vi "Desktop Main.vi"() -> ()   [LabVIEW 2021]
doc: "Demonstrates how to use User Datagram Protocol (UDP) to send data to the myRIO target."
panel:
  in  "LED":bool[](array[boolean])=[FALSE, FALSE, FALSE, FALSE]
  out "error out":errorcluster
  in  "Stop":bool
  in  "Target IP Address":string="172.22.11.2"
  # "Overview: Demonstrates how to use User Datagram Protocol (UDP) to send data to the myRIO target.\nInstructions:\n1. Verify if the value of Target IP Address is correct. If not, specify the correct value.\n2. Run this VI.\n3. Open RT Main.vi and follow its front panel instructions.\n4. Change the value of LED on this VI and observe the value of LED Status on RT Main.vi.\n5. Click Stop to stop this VI."
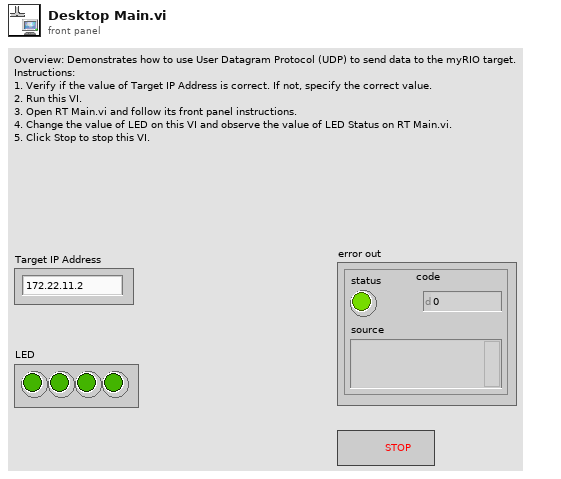
[diagram p1: front panel]
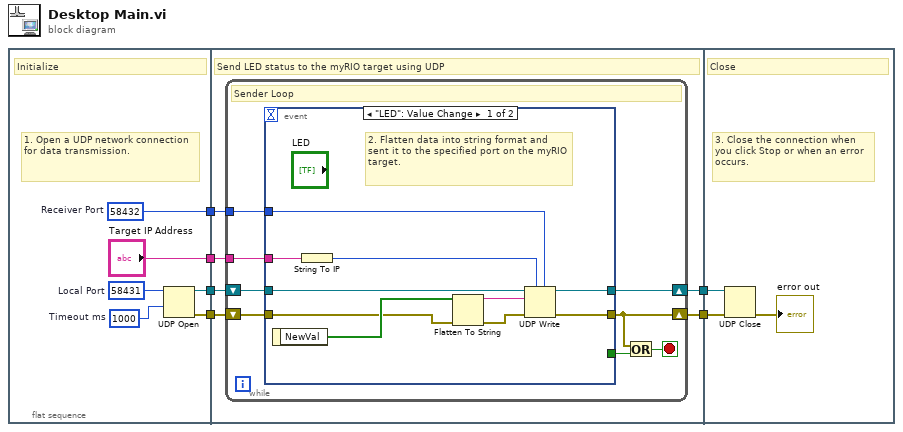
[diagram p0: block diagram]
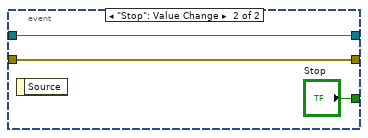
[diagram p2: hidden frame]
diagram:
  n1 = flat-sequence {
    tunnel: [w11] -> w4
    tunnel: [w10] -> w3
    tunnel: ["Target IP Address"] -> w2
    tunnel: [w8] -> w1
    tunnel: [w18] -> w6
    tunnel: [w17] -> w5
    tunnel: w4 -> [w16]
    tunnel: w3 -> [w15]
    tunnel: w2 -> [w14]
    tunnel: w1 -> [w13]
    tunnel: w6 -> [w41]
    tunnel: w5 -> [w42]
    frame #0 {
      w7 = 1000  # Timeout ms
      w8 = u16 58432  # Receiver Port
      w12 = u16 58431  # Local Port
      # "1. Open a UDP network connection for data transmission."
      # "Initialize"
      n2 = UDP Open(9:w7, 11:w12) -> (port=w11:refnum<k16>, 0:w10:errorcluster)  [unwired: 3 in, 1 out]
    }
    frame #1 {
      # "Send LED status to the myRIO target using UDP"
      n3 = while {
        shift-right: [w22] -> w18
        shift-left: w15 -> [w24]
        shift-right: [w25] -> w17
        shift-left: w16 -> [w26]
        tunnel: w14 -> [w20]
        tunnel: w13 -> [w19]
        stop <- w23 stop-if-true
        # "Sender Loop"
        n4 = event shown="[0] \"LED\": Value Change" {
          selector: _ -> [_ _]
          dyn-events: _ -> [_ _]
          timeout: _ -> [_ _]
          tunnel: w26 -> [w33 w38]
          tunnel: [w30 w38] -> w25
          tunnel: w24 -> [w31 w37]
          tunnel: [w29 w37] -> w22
          tunnel: [_ "Stop"] -> w21
          tunnel: w20 -> [w28 _]
          tunnel: w19 -> [w27 _]
          event "LED": Value Change {
            # "2. Flatten data into string format and\nsent it to the specified port on the myRIO target."
            n5 = event-data() -> ("NewVal"=w32:bool[])  [unwired: 1 in]
            n6 = String To IP(1:w28) -> (0:w36:u32)
            n7 = Flatten To String(anything=w32, error in (no error)=w31) -> (data string=w35:string, error out=w34:errorcluster)  [unwired: 2 in, 1 out]
            n8 = UDP Write(address=w36, port or service name=w27, connection ID=w33, data in=w35, 8:w34) -> (error out=w29:errorcluster, 3:w30:refnum<k16>)  [unwired: 1 in]
          }
          event "Stop": Value Change {
            n9 = event-data() -> ()  [unwired: 1 in, 1 out]
          }
        }
        n10 = Or(x=w22, y=w21) -> (x .or. y?=w23:bool)
      }
    }
    frame #2 {
      # "3. Close the connection when you click Stop or when an error occurs."
      # "Close"
      n11 = UDP Close(connection ID=w42, 8:w41) -> (error out=→"error out":errorcluster)  [unwired: 1 out]
    }
  }
